vi "Utility - Display Error for Variant.vi"(8 "error in (no error)":errorcluster, 10 "Step":string) -> (0 "error out":errorcluster)   [LabVIEW 2014]
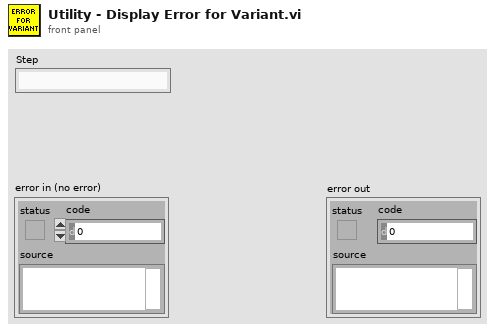
[diagram p1: front panel]
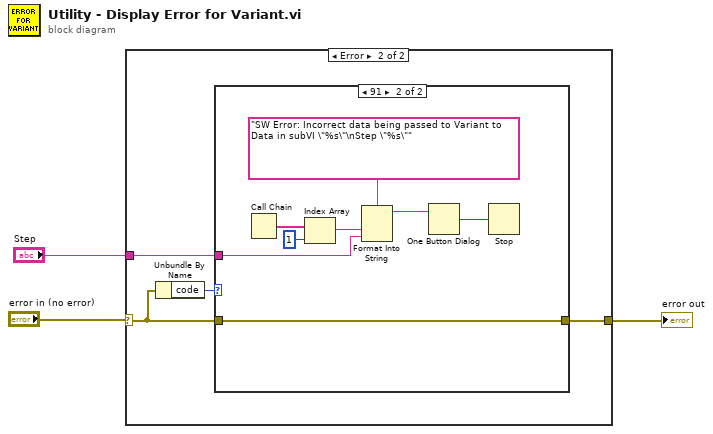
[diagram p0: block diagram]
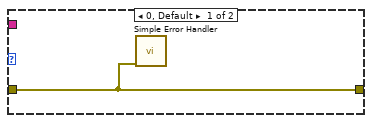
[diagram p3: hidden frame]
diagram:
  n1 = case shown="Error" "error in (no error)" {
    selector: "error in (no error)" -> [w4 w6]
    tunnel: [w4 w7] -> w2
    tunnel: "Step" -> [_ w5]
    frame No Error {
    }
    frame Error {
      n2 = Unbundle By Name(w6) -> ("code"=w8:i32)
      n3 = case shown="91" w8 {
        tunnel: [w9 w17] -> w7
        tunnel: w6 -> [w9 w17]
        tunnel: w5 -> [_ w10]
        frame 0, Default {
          n4 = call <vilib>:"Simple Error Handler.vi"("error in (no error)"=w9) -> ()  [unwired: 4 in, 5 out]
        }
        frame 91 {
          n5 = Call Chain() -> (call chain=w15:string[])
          n6 = Index Array(array=w15, index=1) -> (element=w14:string)
          n7 = Format Into String(format string="SW Error: Incorrect data being passed to Variant to Data in subVI \"%s\"\nStep \"%s\"" ("message"), w14, w10) -> (resulting string=w13:string)  [unwired: 2 in, 1 out]
          n8 = One Button Dialog(message=w13) -> (true=w16:bool)  [unwired: 1 in]
          n9 = Stop(stop? (T)=w16) -> ()
        }
      }
    }
  }
  "error out" <- w2
